vi "Is GUI Running - Set.vi"(0 "Is GUI Running?":bool) -> ()   [LabVIEW 2023, in "Error Manager.lvlib" / "New Error Dialogue GUI.lvlib"]
uses:
  New Error Dialogue GUI.lvlib
  Is GUI Running (library variable).vi
panel:
  # "Development\ncontrols/indicators useful for development and testing, but which are not outputs of the VI"
  # "Input\nInputs to the VI"
  # "Output\nOutputs of the VI"
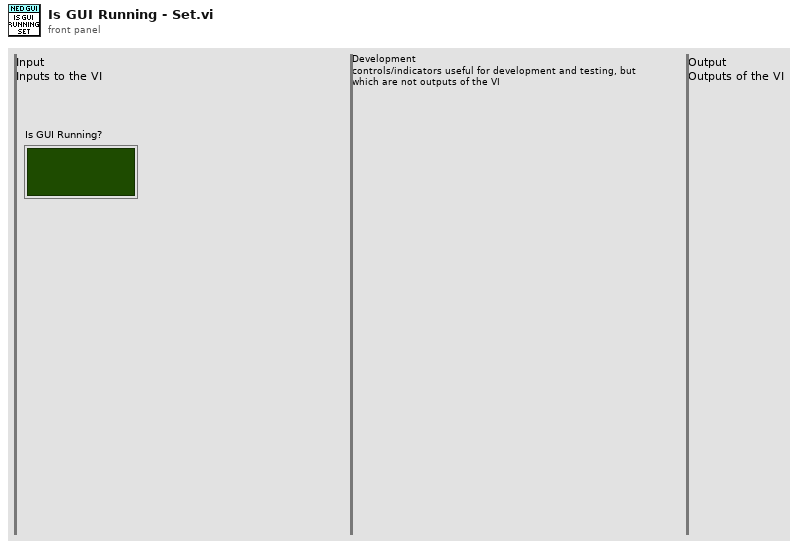
[diagram p1: front panel]
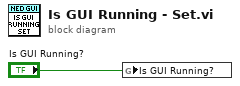
[diagram p0: block diagram]
diagram:
  n1 = global write "Is GUI Running (library variable).vi" "Is GUI Running?"("Is GUI Running?") -> ()
